vi "SeimensS7Net_OperateResult.vi"(8 "error in (no error)":errorcluster caption="错误输入（无错误）", 11 "OperateResult":refnum<k24>) -> (0 "error out":errorcluster caption="错误输出")   [LabVIEW 2018, in "Seimens.lvclass"]
uses:
  Seimens.lvclass
  D:/LiMing/Labview/lib/LM_HslCommunication/DLL/HslCommunication.dll
  DLL/HslCommunication.dll
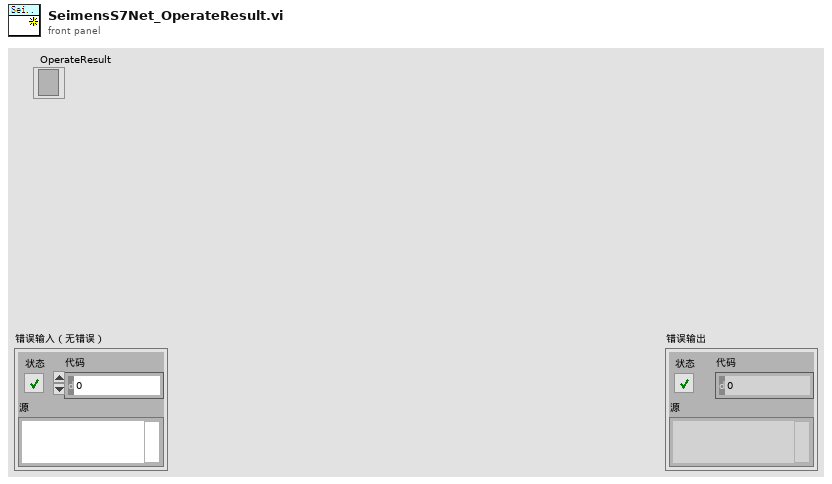
[diagram p1: front panel]
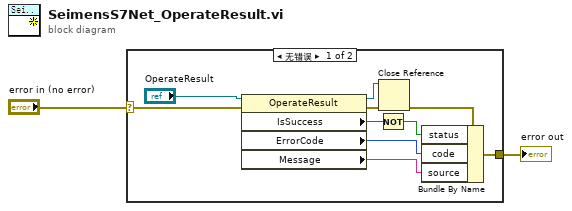
[diagram p0: block diagram]
diagram:
  n1 = case shown="无错误" "error in (no error)" {
    selector: "error in (no error)" -> [w9 w13]
    tunnel: [w6 w13] -> w1
    frame No Error {
      n2 = property class="OperateResult"(reference="OperateResult", error in=w9) -> (reference out=w11:refnum<k24>, error out=w12:errorcluster, "IsSuccess"=w4:bool, "ErrorCode"=w5:i32, "Message"=w8:string)
      n3 = Not(x=w4) -> (.not. x?=w3:bool)
      n4 = Close Reference(reference=w11, error in (no error)=w12) -> (error out=w7:errorcluster)
      n5 = Bundle By Name(cluster=w7, "status"=w3, "code"=w5, "source"=w8) -> (w6:errorcluster)
    }
    frame Error {
    }
  }
  "error out" <- w1
